vi "testParseStateQueueTimeoutHandling.vi"(8 "error in (no error)":errorcluster, 11 "testStateMachineUtilities in":refnum<class "testStateMachineUtilities.lvclass">) -> (0 "error out":errorcluster, 3 "testStateMachineUtilities out":refnum<class "testStateMachineUtilities.lvclass">)   [LabVIEW 2013, in "testStateMachineUtilities.lvclass"]
uses:
  testStateMachineUtilities.lvclass
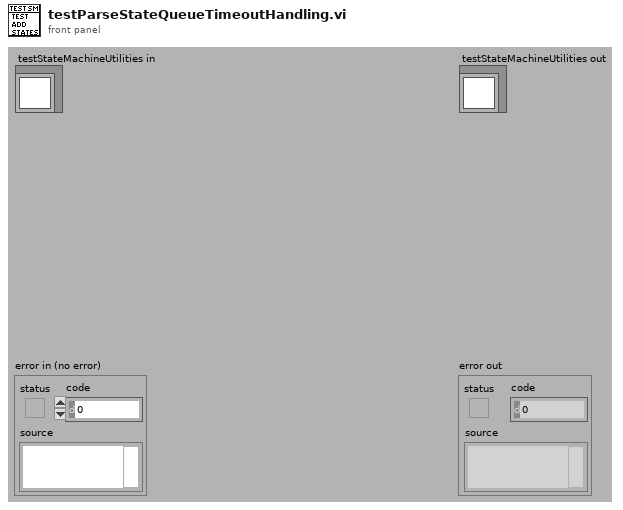
[diagram p1: front panel]
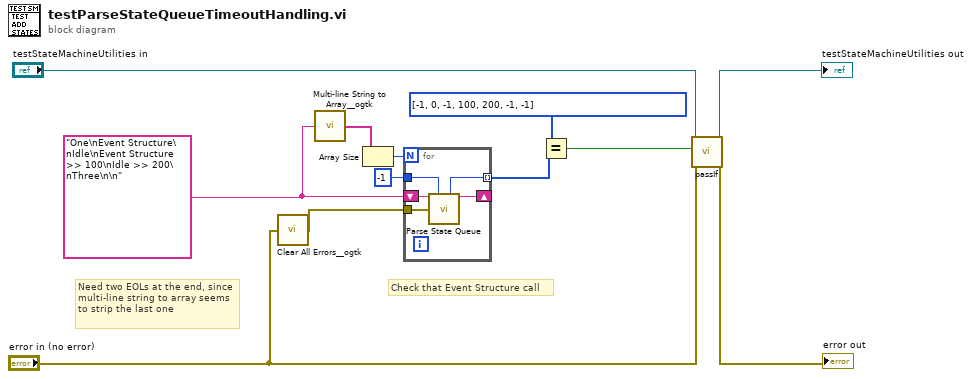
[diagram p0: block diagram]
diagram:
  w7 = "One\nEvent Structure\nIdle\nEvent Structure >> 100\nIdle >> 200\nThree\n\n" ("State Queue")
  # "Need two EOLs at the end, since multi-line string to array seems to strip the last one"
  # "Check that Event Structure call"
  n1 = call <userlib>:"Clear All Errors__ogtk.vi"("Error In"="error in (no error)") -> ("Error Out"=w8:errorcluster)  [unwired: 3 in]
  n2 = call <userlib>:"Multi-line String to Array__ogtk.vi"("string"=w7) -> ("lines"=w5:string[])
  n3 = Array Size(array=w5) -> (size(s)=w6:i32)
  n4 = for {
    N: w6 -> [_]
    tunnel: w8 -> [w16]
    shift-right: [w15] -> _
    shift-left: w7 -> [w17]
    tunnel: -1 ("Timeout") -> [w14]
    tunnel: [w13] -> w2 mode=indexing
    n5 = call "Parse State Queue.vi"("State Queue"=w17, "Timeout"=w14, "Error In (no error)"=w16) -> ("Timeout out"=w13:i32, "Remaining States"=w15:string)  [unwired: 9 in, 2 out]
  }
  n6 = Equal?(x=i32[] [-1, 0, -1, 100, 200, -1, -1] ("Array"), y=w2) -> (x = y?=w1:bool)
  n7 = call-dynamic "passIf.vi"("error in (no error)"="error in (no error)", "pass"=w1, "TestCase in"="testStateMachineUtilities in") -> ("error out"=→"error out":errorcluster, "TestCase out"=→"testStateMachineUtilities out":refnum<class "testStateMachineUtilities.lvclass">)  [unwired: 7 in]
